vi "Add Channel to All Transfers.vi"(7 "GUID (Default Channel)":string="03D3BB99-1485-13A6-561D1F898F032919", 8 "error in (no error)":errorcluster, 9 "Channel":T1, 10 "Channel Name":string, 11 "Item Ref in":T3 format="%.0x") -> (0 "error out":errorcluster, 3 "Item Ref out":T3 format="%.0x")   [LabVIEW 2017, in "DSF System Explorer.lvlib"]
uses:
  DSF System Explorer.lvlib
  <vilib>/NI Veristand/Custom Device API/Custom Device Item Ref.ctl
  <vilib>/NI Veristand/Custom Device API/Custom Device Channel.ctl
  <vilib>/NI Veristand/Custom Device API/Custom Device Channel Type.ctl
  <vilib>/NI Veristand/Custom Device API/Custom Device API.lvlib
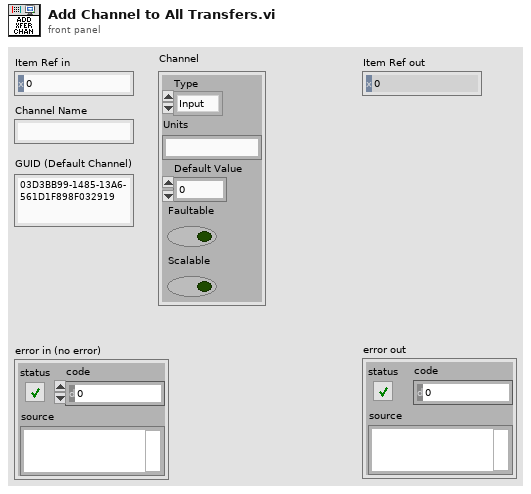
[diagram p1: front panel]
types:
  T1 = typedef "Custom Device API.lvlib/Custom Device Channel.ctl" = cluster{"Type":T2, "Units":string, "Default Value":dbl, "Faultable":bool, "Scalable":bool}
  T2 = typedef "Custom Device API.lvlib/Custom Device Channel Type.ctl" = enum16{"Input", "Output"}
  T3 = typedef "Custom Device API.lvlib/Custom Device Item Ref.ctl" = u64
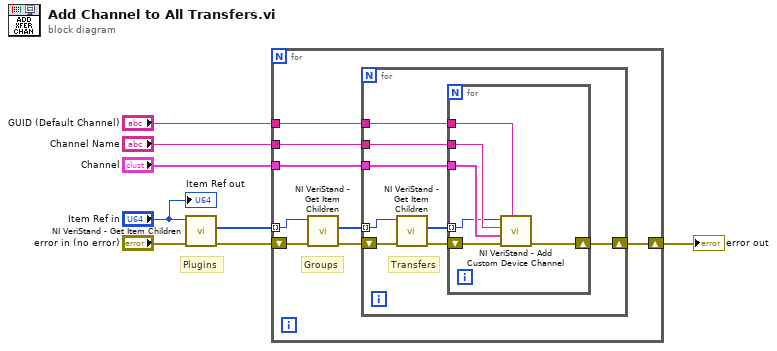
[diagram p0: block diagram]
diagram:
  # "Plugins"
  n1 = call <vilib>:"NI VeriStand - Get Item Children.vi"("error in (no error)"="error in (no error)", "Item Ref in"="Item Ref in") -> ("error out"=w6:errorcluster, "Child Refs"=w5:T3[])  [unwired: 6 in, 2 out]
  n2 = for {
    shift-right: [w13] -> w4
    shift-left: w6 -> [w16]
    tunnel: w5 -> [w15] mode=indexing
    tunnel: "Channel Name" -> [w11]
    tunnel: "Channel" -> [w10]
    tunnel: "GUID (Default Channel)" -> [w9]
    # "Groups"
    n3 = call <vilib>:"NI VeriStand - Get Item Children.vi"("error in (no error)"=w16, "Item Ref in"=w15) -> ("error out"=w14:errorcluster, "Child Refs"=w12:T3[])  [unwired: 6 in, 2 out]
    n4 = for {
      shift-right: [w24] -> w13
      shift-left: w14 -> [w23]
      tunnel: w12 -> [w21] mode=indexing
      tunnel: w11 -> [w19]
      tunnel: w10 -> [w20]
      tunnel: w9 -> [w18]
      # "Transfers"
      n5 = call <vilib>:"NI VeriStand - Get Item Children.vi"("error in (no error)"=w23, "Item Ref in"=w21) -> ("error out"=w22:errorcluster, "Child Refs"=w17:T3[])  [unwired: 6 in, 2 out]
      n6 = for {
        shift-right: [w29] -> w24
        shift-left: w22 -> [w30]
        tunnel: w20 -> [w28]
        tunnel: w19 -> [w27]
        tunnel: w18 -> [w26]
        tunnel: w17 -> [w25] mode=indexing
        n7 = call <vilib>:"NI VeriStand - Add Custom Device Channel.vi"("GUID (Default Channel)"=w26, "error in (no error)"=w30, "Channel"=w28, "Channel Name"=w27, "Parent Ref in"=w25) -> ("error out"=w29:errorcluster)  [unwired: 3 in, 3 out]
      }
    }
  }
  "error out" <- w4
  "Item Ref out" <- "Item Ref in"
